vi "Initialize Routing Channel Page (State Configuration).vi"(8 "error in (no error)":errorcluster, 9 "Alias Mappings":T1[](array[typedef]), 10 "Routing Channel Page Controls":T3, 11 "Routing Channel Ref in":T4 format="%.0x") -> (0 "error out":errorcluster, 3 "Routing Channel Ref out":T4 format="%.0x")   [LabVIEW 2020, in "Routing and Faulting System Explorer.lvlib"]
uses:
  Routing and Faulting System Explorer.lvlib
  <vilib>/NI VeriStand/Custom Device API/Custom Device Item Ref.ctl
  Routing Channel Page Controls.ctl
  Shared/Alias Mapping.ctl
  Shared/Alias Endpoint.ctl
  Shared/Constants.vi
  Scripting/Routing and Faulting Scripting.lvlib
  Shared/Routing and Faulting Shared.lvlib
  <vilib>/NI VeriStand/Custom Device API/Custom Device API.lvlib
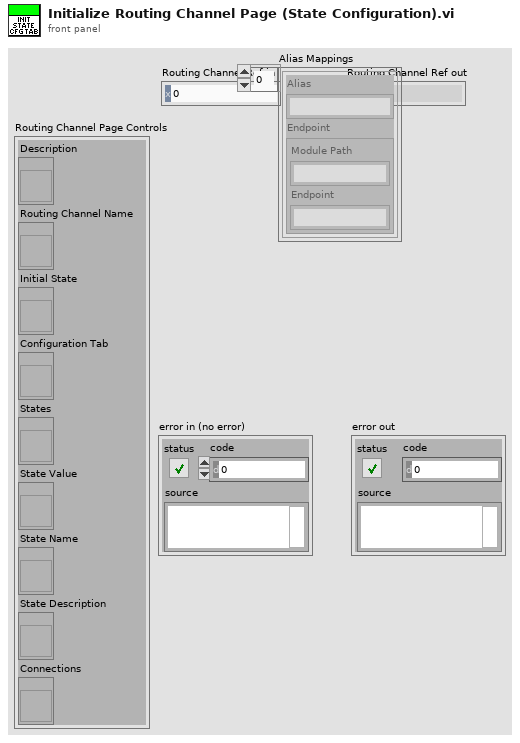
[diagram p1: front panel]
types:
  T1 = typedef "Routing and Faulting Shared.lvlib/Alias Mapping.ctl" = cluster{"Alias":string, "Endpoint":T2}
  T2 = typedef "Routing and Faulting Shared.lvlib/Alias Endpoint.ctl" = cluster{"Module Path":string, "Endpoint":string}
  T3 = typedef "Routing and Faulting System Explorer.lvlib/Routing Channel Page Controls.ctl" = cluster{"Description":refnum<vi>, "Routing Channel Name":refnum<vi>, "Initial State":refnum<vi>, "Configuration Tab":refnum<vi>, "States":refnum<vi>, "State Value":refnum<vi>, "State Name":refnum<vi>, "State Description":refnum<vi>, "Connections":refnum<vi>}
  T4 = typedef "Custom Device API.lvlib/Custom Device Item Ref.ctl" = u64
  T5 = enum8{"Enabled", "Disabled", "Disabled and Grayed Out"}
  T6 = typedef "Routing and Faulting Shared.lvlib/Routing State.ctl" = cluster{"Name":string, "Description":string, "Value":i32, "Connection List":T7[]}
  T7 = typedef "Routing and Faulting Shared.lvlib/Connection.ctl" = cluster{"Module":string, "Source":string, "Destination":string}
  T8 = typedef "Routing and Faulting System Explorer.lvlib/Connection Row.ctl" = cluster{"Source":string, "Destination":string, "Edit":bool, "Remove":bool}
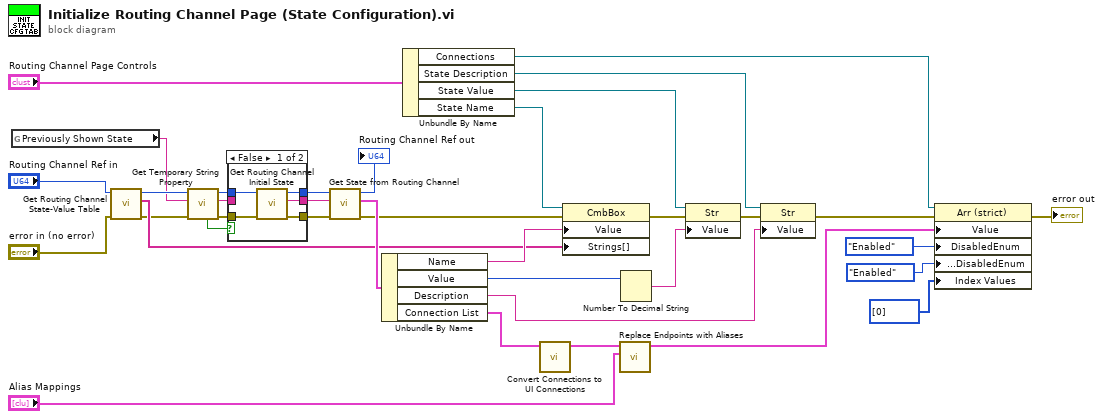
[diagram p0: block diagram]
diagram:
  n1 = global read "Constants.vi" "Previously Shown State"() -> (w2:string)
  n2 = call "Get Routing Channel State-Value Table.vi"("error in"="error in (no error)", "routing channel in"="Routing Channel Ref in") -> ("error out"=w8:errorcluster, "state names"=w14:string[], "routing channel out"=w7:T4)  [unwired: 6 in, 1 out]
  n3 = call "Get Temporary String Property.vi"("error in (no error)"=w8, "property name"=w2, "Item Ref in"=w7) -> ("error out"=w6:errorcluster, "value"=w4:string, "Item Ref out"=w3:T4, "found?"=w5:bool)  [unwired: 5 in]
  n4 = case shown="False" w5 {
    tunnel: [w41 w43] -> w34
    tunnel: [w40 w42] -> w21
    tunnel: [w39 w44] -> w20
    tunnel: w6 -> [w38 w44]
    tunnel: w4 -> [_ w43]
    tunnel: w3 -> [w37 w42]
    frame False {
      n5 = call "Get Routing Channel Initial State.vi"("error in"=w38, "routing channel in"=w37) -> ("error out"=w39:errorcluster, "initial state"=w41:string, "routing channel out"=w40:T4)  [unwired: 7 in]
    }
    frame True {
    }
  }
  n6 = call "Get State from Routing Channel.vi"("error in"=w20, "state"=w34, "routing channel in"=w21) -> ("error out"=w32:errorcluster, "state and connections"=w33:T6, "routing channel out"=→"Routing Channel Ref out":T4)  [unwired: 6 in]
  n7 = Unbundle By Name(w33) -> ("Name"=w31:string, "Value"=w29:i32, "Description"=w16:string, "Connection List"=w19:T7[])
  n8 = Unbundle By Name("Routing Channel Page Controls") -> ("Connections"=w1:refnum<vi>, "State Description"=w17:refnum<vi>, "State Value"=w26:refnum<vi>, "State Name"=w15:refnum<vi>)
  n9 = call "Convert Connections to UI Connections.vi"("Connection List"=w19) -> ("UI Connections List"=w12:T8[])  [unwired: 10 in]
  n10 = property class="CmbBox"(reference=w15, error in=w32, "Value"=w31, "Strings[]"=w14) -> (error out=w30:errorcluster)  [unwired: 1 out]
  n11 = call "Replace Endpoints with Aliases.vi"("Alias Mappings"="Alias Mappings", "UI Connections List in"=w12) -> ("UI Connections List out"=w11:T8[])  [unwired: 9 in]
  n12 = Number To Decimal String(number=w29) -> (decimal integer string=w28:string)  [unwired: 1 in]
  n13 = property class="Str"(reference=w26, error in=w30, "Value"=w28) -> (error out=w18:errorcluster)  [unwired: 1 out]
  n14 = property class="Str"(reference=w17, error in=w18, "Value"=w16) -> (error out=w13:errorcluster)  [unwired: 1 out]
  n15 = property class="Arr (strict)"(reference=w1, error in=w13, "Value"=w11, "DisabledEnum"=T5."Enabled" ("Disabled"), "Array Element.DisabledEnum"=T5."Enabled" ("Array Element.Disabled"), "Index Values"=u32[] [0]) -> (error out=→"error out":errorcluster)  [unwired: 1 out]
